vi "create data dictionary from collection.vi"(8 "error in":errorcluster, 11 "tag collection":refnum<class "data bus tag collection.lvclass">) -> (0 "error out":errorcluster, 3 "data dictionary":refnum<class "data bus dictionary.lvclass">)   [LabVIEW 2013, in "data bus dictionary.lvclass"]
doc: "Accepts a set of tag descriptors and generates a fully formed data dictionary from these tags."
uses:
  data bus dictionary.lvclass
  tag collection/data bus tag collection.lvclass
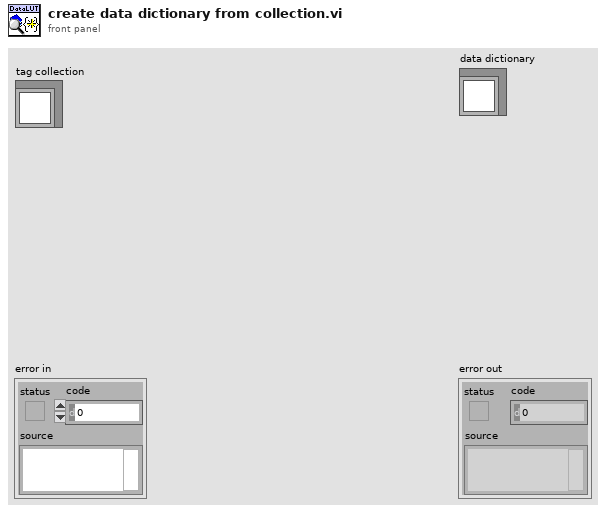
[diagram p1: front panel]
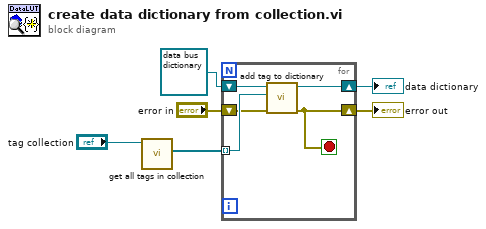
[diagram p0: block diagram]
diagram:
  n1 = call "get all tags in collection.vi"("tag collection in"="tag collection") -> ("tags"=w1:refnum<class "data bus tag description.lvclass">[])  [unwired: 8 in, 2 out]
  n2 = for {
    shift-right: [w7] -> w3
    shift-left: "error in" -> [w9]
    shift-right: [w8] -> w4
    shift-left: refnum<class "data bus dictionary.lvclass"> refnum ("Data Locator in") -> [w11]
    tunnel: w1 -> [w10] mode=indexing
    stop <- w7 stop-if-true
    n3 = call "add tag to dictionary.vi"("error in"=w9, "system tag"=w10, "data dictionary in"=w11) -> ("error out"=w7:errorcluster, "data dictionary out"=w8:refnum<class "data bus dictionary.lvclass">)  [unwired: 7 in]
  }
  "error out" <- w3
  "data dictionary" <- w4
